vi "Sub-sample Timing Offset.vi"(9 "Sample Offset":i32, 11 "output complex waveform in":T1 caption="output complex waveform" {"Y" format="%.3f"; "dt" format="%^.2e"; "t0" format="%.4f"}) -> (3 "output complex waveform out":T1 caption="output complex waveform" {"Y" format="%.3f"; "dt" format="%^.2e"; "t0" format="%.4f"})   [LabVIEW 2012]
uses:
  <vilib>/addons/Modulation/Analog/controls/Complex Data Waveform.ctl
  <vilib>/addons/Modulation/niAMT.lvlib
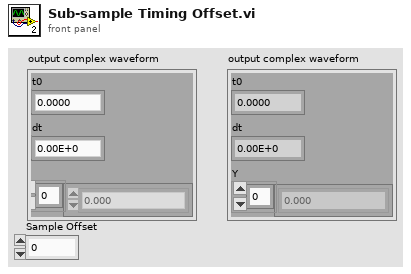
[diagram p1: front panel]
types:
  T1 = typedef "niAMT.lvlib/Complex Data Waveform.ctl" = cluster{"t0":dbl, "dt":dbl, "Y":cdb[]}
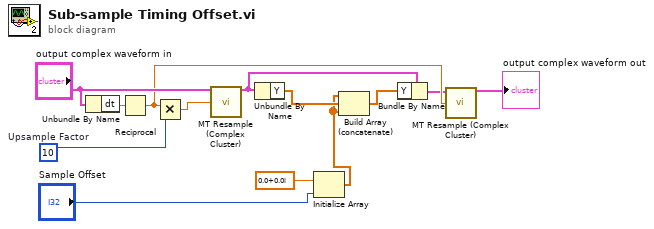
[diagram p0: block diagram]
diagram:
  w11 = 10  # Upsample Factor
  n1 = Unbundle By Name("output complex waveform in") -> ("dt"=w12:dbl)
  n2 = Reciprocal(x=w12) -> (1/x=w8:dbl)
  n3 = Multiply(x=w8, y=w11) -> (x*y=w10:dbl)
  n4 = call <vilib>:"MT Resample (Complex Cluster).vi"("input complex waveform"="output complex waveform in", "desired sample rate (Hz)"=w10) -> ("output complex waveform"=w6:T1)  [unwired: 12 in, 1 out]
  n5 = Unbundle By Name(w6) -> ("Y"=w5:cdb[])
  n6 = Initialize Array(cdb 0.0+0.0i ("Numeric"), "Sample Offset") -> (w1:cdb[])
  n7 = Build Array (concatenate)(w1, w5, w1) -> (w2:cdb[])
  n8 = Bundle By Name(cluster=w6, "Y"=w2) -> (w7:T1)
  n9 = call <vilib>:"MT Resample (Complex Cluster).vi"("input complex waveform"=w7, "desired sample rate (Hz)"=w8) -> ("output complex waveform"=→"output complex waveform out":T1)  [unwired: 12 in, 1 out]
